vi "FGV - System Directories.vi"(7 "FGV State":T1, 8 "error in (no error)":errorcluster, 11 "Path In":path) -> (0 "error out":errorcluster, 2 "System Directory Out":path, 3 "Path Out":path)   [LabVIEW 2021, in "Path Utilities.lvlib"]
doc: "FGV for \"System Directories\" VIs."
uses:
  Path Utilities.lvlib
  TypeDefs/FGV State - System Directories.ctl
  TypeDefs/FGV Data - System Directories.ctl
  <vilib>/Utility/sysdir.llb/System Directory Type.ctl
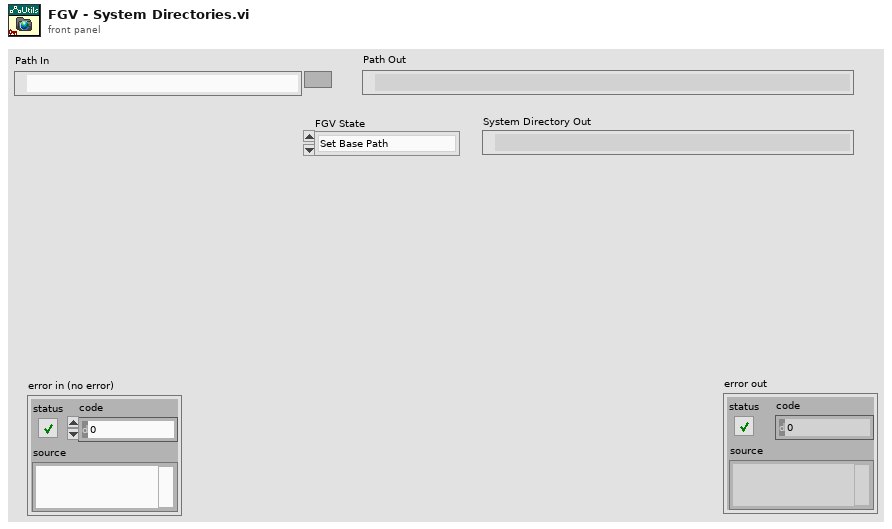
[diagram p1: front panel]
types:
  T1 = typedef "Path Utilities.lvlib/FGV State - System Directories.ctl" = enum16{"Set Base Path", "Get Program Files", "Get Program Data", "Get App Data Local", "Get App Data Roaming", "Get User Documents", "Get Public Documents"}
  T2 = typedef "Path Utilities.lvlib/FGV Data - System Directories.ctl" = cluster{"Base Path":path}
  T3 = typedef "System Directory Type.ctl" = i32
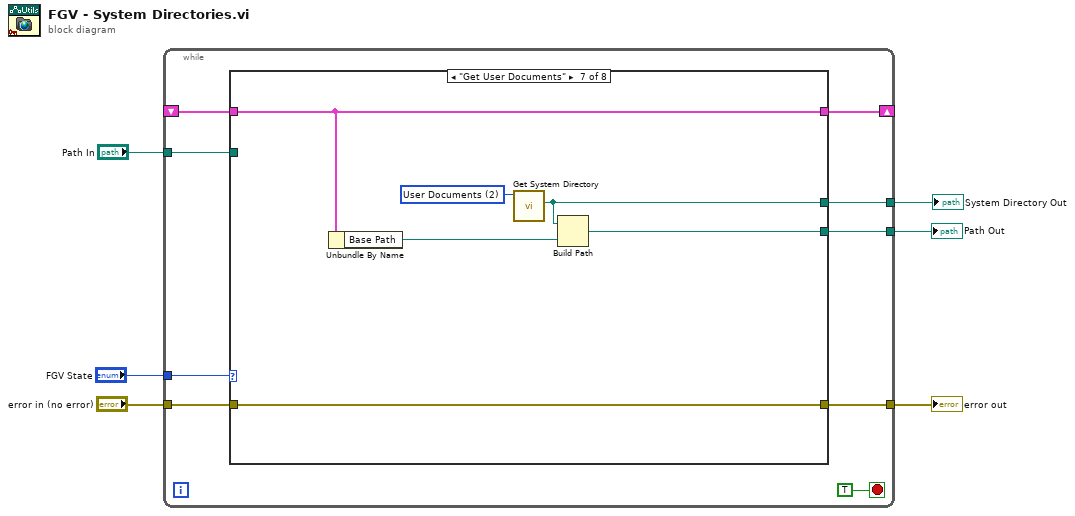
[diagram p0: block diagram]
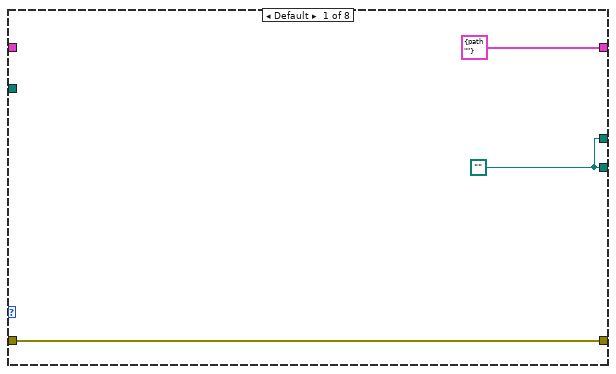
[diagram p2: hidden frame]
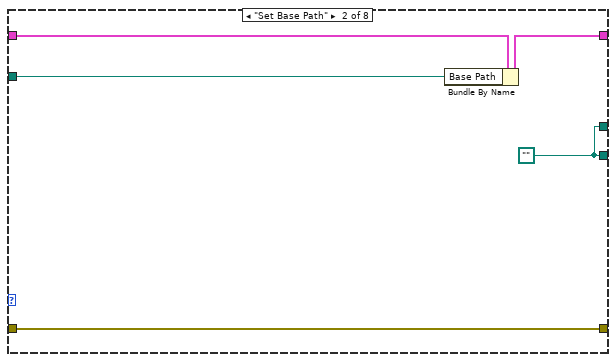
[diagram p3: hidden frame]
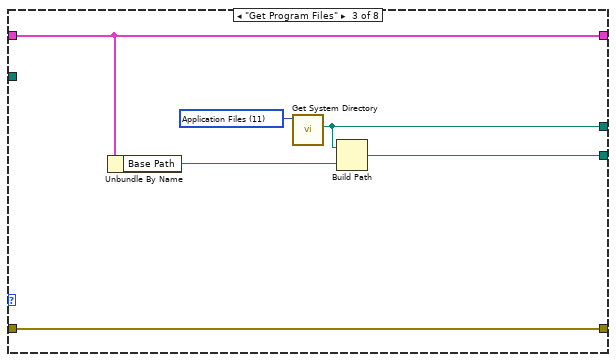
[diagram p4: hidden frame]
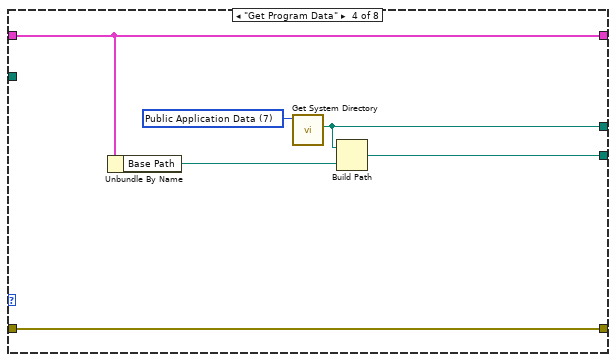
[diagram p5: hidden frame]
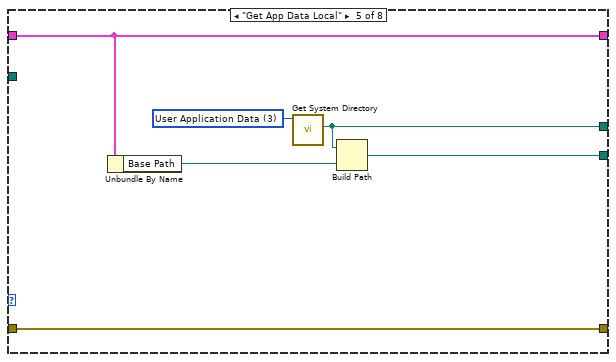
[diagram p6: hidden frame]
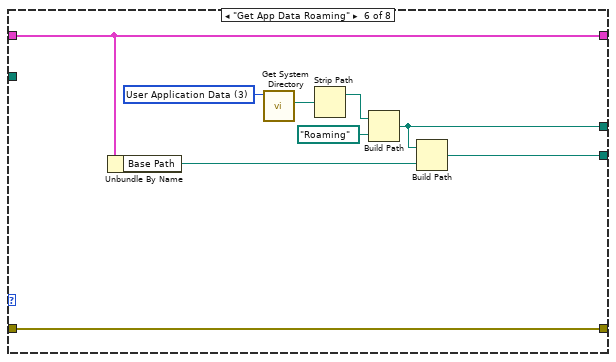
[diagram p7: hidden frame]
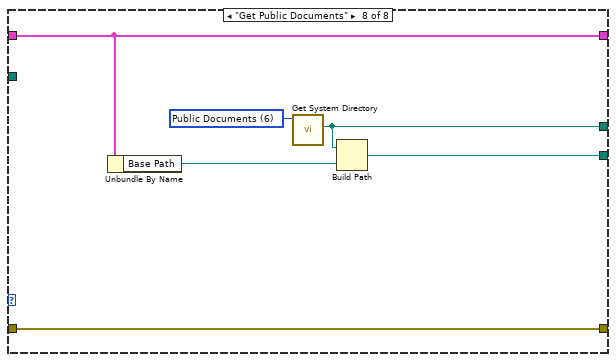
[diagram p8: hidden frame]
diagram:
  n1 = while {
    shift-right: [w11] -> _
    shift-left: _ -> [w9]
    tunnel: "FGV State" -> [w14]
    tunnel: "error in (no error)" -> [w13]
    tunnel: [w12] -> w4
    tunnel: "Path In" -> [w10]
    tunnel: [w8] -> w2
    tunnel: [w7] -> w1
    stop <- TRUE stop-if-true
    n2 = case shown="\"Get User Documents\"" w14 {
      tunnel: w13 -> [w17 w23 w25 w31 w37 w46 w52 w58]
      tunnel: [w17 w23 w25 w31 w37 w46 w52 w58] -> w12
      tunnel: [T2 {"Base Path"=path ""} ("FGV Data") w22 w28 w34 w40 w49 w55 w61] -> w11
      tunnel: w10 -> [_ w21 _ _ _ _ _ _]
      tunnel: w9 -> [_ w20 w28 w34 w40 w49 w55 w61]
      tunnel: [w16 w19 w26 w32 w38 w47 w53 w59] -> w8
      tunnel: [w16 w19 w24 w30 w36 w42 w51 w57] -> w7
      frame Default {
        w16 = path ""
      }
      frame "Set Base Path" {
        w19 = path ""
        n3 = Bundle By Name(cluster=w20, "Base Path"=w21) -> (w22:T2)
      }
      frame "Get Program Files" {
        w29 = T3 11 items=["User Home"=0, "User Desktop"=1, "User Documents"=2, "User Application Data"=3, "User Preferences"=4, "User Temporary"=5, "Public Documents"=6, "Public Application Data"=7, "Public Preferences"=8, "Public Cache"=13, "System Core Libraries"=9, "System Installed Libraries"=10, "Application Files"=11, "Boot Volume Root"=12] ("system directory type")
        n4 = Unbundle By Name(w28) -> ("Base Path"=w27:path)
        n5 = call <vilib>:"Get System Directory.vi"("system directory type"=w29) -> ("system directory"=w24:path)  [unwired: 10 in]
        n6 = Build Path(base path=w24, name or relative path=w27) -> (appended path=w26:path)
      }
      frame "Get Program Data" {
        w35 = T3 7 items=["User Home"=0, "User Desktop"=1, "User Documents"=2, "User Application Data"=3, "User Preferences"=4, "User Temporary"=5, "Public Documents"=6, "Public Application Data"=7, "Public Preferences"=8, "Public Cache"=13, "System Core Libraries"=9, "System Installed Libraries"=10, "Application Files"=11, "Boot Volume Root"=12] ("system directory type")
        n7 = Unbundle By Name(w34) -> ("Base Path"=w33:path)
        n8 = call <vilib>:"Get System Directory.vi"("system directory type"=w35) -> ("system directory"=w30:path)  [unwired: 10 in]
        n9 = Build Path(base path=w30, name or relative path=w33) -> (appended path=w32:path)
      }
      frame "Get App Data Local" {
        w41 = T3 3 items=["User Home"=0, "User Desktop"=1, "User Documents"=2, "User Application Data"=3, "User Preferences"=4, "User Temporary"=5, "Public Documents"=6, "Public Application Data"=7, "Public Preferences"=8, "Public Cache"=13, "System Core Libraries"=9, "System Installed Libraries"=10, "Application Files"=11, "Boot Volume Root"=12] ("system directory type")
        n10 = Unbundle By Name(w40) -> ("Base Path"=w39:path)
        n11 = call <vilib>:"Get System Directory.vi"("system directory type"=w41) -> ("system directory"=w36:path)  [unwired: 10 in]
        n12 = Build Path(base path=w36, name or relative path=w39) -> (appended path=w38:path)
      }
      frame "Get App Data Roaming" {
        w50 = T3 3 items=["User Home"=0, "User Desktop"=1, "User Documents"=2, "User Application Data"=3, "User Preferences"=4, "User Temporary"=5, "Public Documents"=6, "Public Application Data"=7, "Public Preferences"=8, "Public Cache"=13, "System Core Libraries"=9, "System Installed Libraries"=10, "Application Files"=11, "Boot Volume Root"=12] ("system directory type")
        n13 = Unbundle By Name(w49) -> ("Base Path"=w48:path)
        n14 = call <vilib>:"Get System Directory.vi"("system directory type"=w50) -> ("system directory"=w45:path)  [unwired: 10 in]
        n15 = Strip Path(path=w45) -> (stripped path=w44:path)  [unwired: 1 out]
        n16 = Build Path(base path=w44, name or relative path=path "Roaming") -> (appended path=w42:path)
        n17 = Build Path(base path=w42, name or relative path=w48) -> (appended path=w47:path)
      }
      frame "Get User Documents" {
        w56 = T3 2 items=["User Home"=0, "User Desktop"=1, "User Documents"=2, "User Application Data"=3, "User Preferences"=4, "User Temporary"=5, "Public Documents"=6, "Public Application Data"=7, "Public Preferences"=8, "Public Cache"=13, "System Core Libraries"=9, "System Installed Libraries"=10, "Application Files"=11, "Boot Volume Root"=12] ("system directory type")
        n18 = Unbundle By Name(w55) -> ("Base Path"=w54:path)
        n19 = call <vilib>:"Get System Directory.vi"("system directory type"=w56) -> ("system directory"=w51:path)  [unwired: 10 in]
        n20 = Build Path(base path=w51, name or relative path=w54) -> (appended path=w53:path)
      }
      frame "Get Public Documents" {
        w62 = T3 6 items=["User Home"=0, "User Desktop"=1, "User Documents"=2, "User Application Data"=3, "User Preferences"=4, "User Temporary"=5, "Public Documents"=6, "Public Application Data"=7, "Public Preferences"=8, "Public Cache"=13, "System Core Libraries"=9, "System Installed Libraries"=10, "Application Files"=11, "Boot Volume Root"=12] ("system directory type")
        n21 = Unbundle By Name(w61) -> ("Base Path"=w60:path)
        n22 = call <vilib>:"Get System Directory.vi"("system directory type"=w62) -> ("system directory"=w57:path)  [unwired: 10 in]
        n23 = Build Path(base path=w57, name or relative path=w60) -> (appended path=w59:path)
      }
    }
  }
  "error out" <- w4
  "Path Out" <- w2
  "System Directory Out" <- w1
